vi "CheckConnectivity.vi"(8 "error in (no error)":errorcluster, 11 "SensorBase in":refnum<class "SensorBase.lvclass">) -> (0 "error out":errorcluster, 2 "Are any Connected?":bool, 3 "SensorBase out":refnum<class "SensorBase.lvclass">)   [LabVIEW 2018, in "SensorPlugins.lvlib" / "SensorBase.lvclass"]
doc: "This VI checks if communication has been sucessfully established between software and the instrument."
uses:
  SensorBase.lvclass
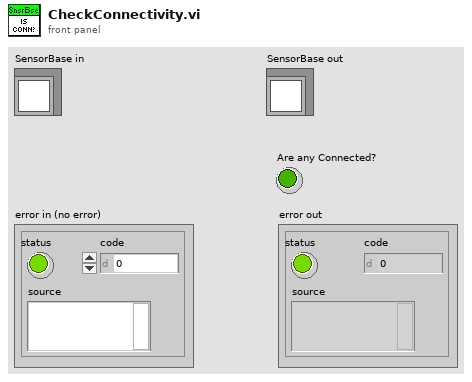
[diagram p1: front panel]
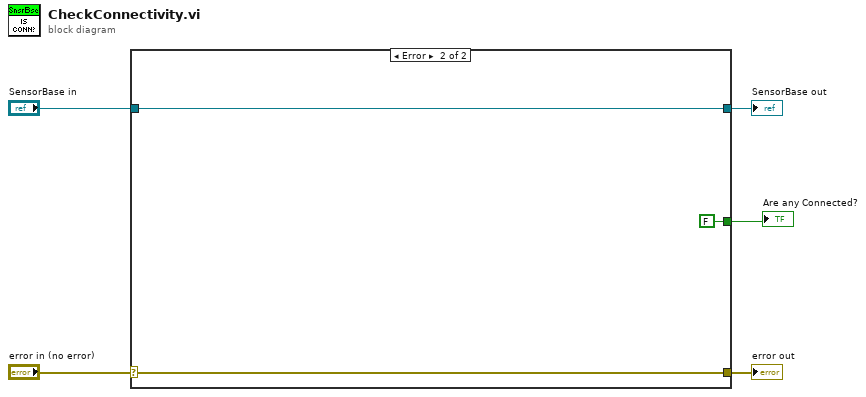
[diagram p0: block diagram]
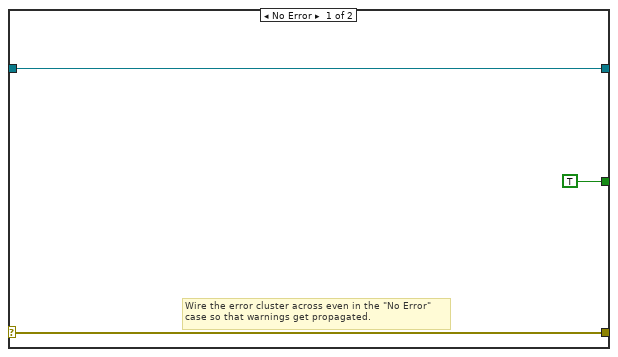
[diagram p2: hidden frame]
diagram:
  n1 = case shown="Error" "error in (no error)" {
    selector: "error in (no error)" -> [w7 w11]
    tunnel: [w7 w11] -> w4
    tunnel: [w8 w10] -> w2
    tunnel: "SensorBase in" -> [w8 w10]
    tunnel: [TRUE ("Are any Connected?") FALSE ("Are any Connected?")] -> w1
    frame No Error {
      # "Wire the error cluster across even in the \"No Error\"\ncase so that warnings get propagated."
    }
    frame Error {
    }
  }
  "error out" <- w4
  "SensorBase out" <- w2
  "Are any Connected?" <- w1
